vi "SendCommand_RetrieveResponse.vi"(8 "error in (no error)":errorcluster, 9 "Timeout (Seconds)":dbl=5.0 caption="Time Target (s)", 10 "Input Command":string, 11 "VISA Input":refnum<visa-resource-name>) -> (0 "error out":errorcluster, 1 "Timeout?":bool, 2 "System Response":string, 3 "VISA Output":refnum<visa-resource-name>)   [LabVIEW 2015]
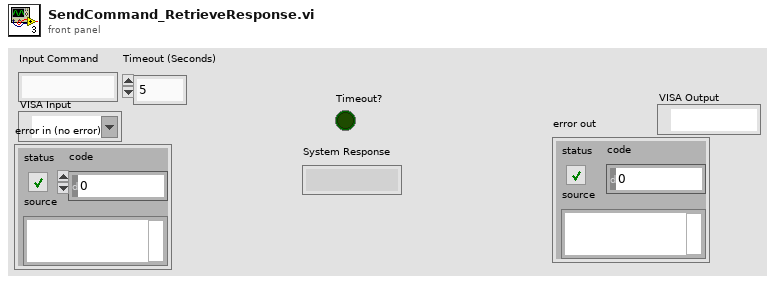
[diagram p1: front panel]
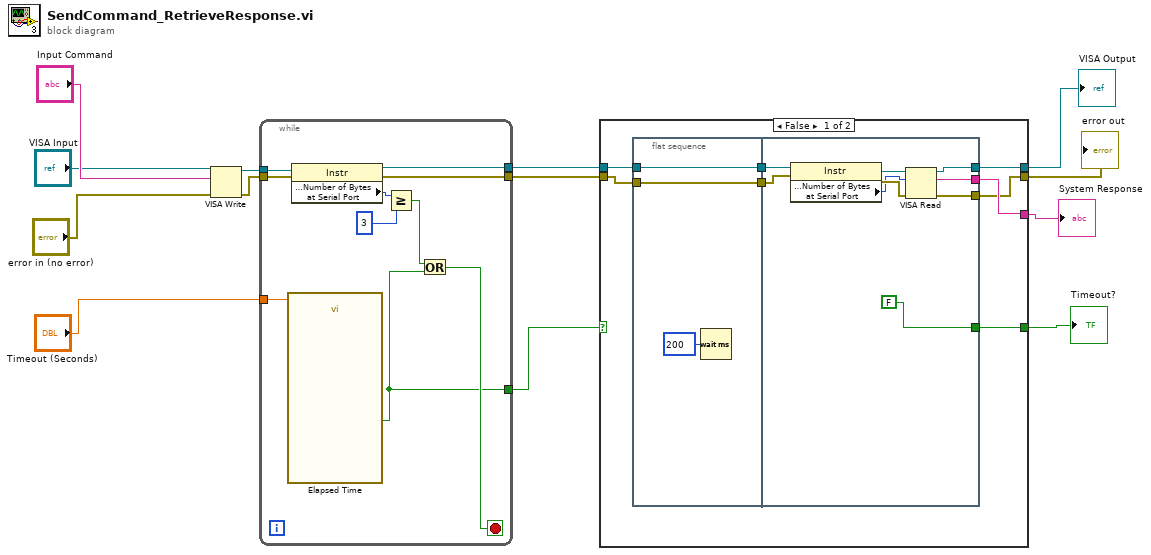
[diagram p0: block diagram]
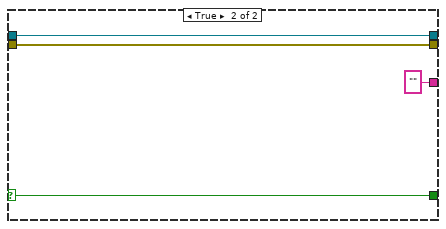
[diagram p2: hidden frame]
diagram:
  n1 = VISA Write(VISA resource name="VISA Input", write buffer="Input Command", error in (no error)="error in (no error)") -> (VISA resource name out=w13:refnum<visa-resource-name>, error out=w12:errorcluster)  [unwired: 1 out]
  n2 = while {
    tunnel: w13 -> [w23]
    tunnel: w12 -> [w22]
    tunnel: [w21] -> w6
    tunnel: [w20] -> w5
    tunnel: "Timeout (Seconds)" -> [w18]
    tunnel: [w15] -> w7
    stop <- w16 stop-if-true
    n3 = call "Elapsed Time"("Time Target (s)"=w18) -> ("Time has Elapsed"=w15:bool)  [unwired: 11 in, 7 out]
    n4 = property class="Instr"(reference=w23, error in=w22) -> (reference out=w21:refnum<visa-resource-name>, error out=w20:errorcluster, "Serial Settings:Number of Bytes at Serial Port"=w14:u32)
    n5 = Greater Or Equal?(x=w14, y=u32 3) -> (x >= y?=w17:bool)
    n6 = Or(x=w17, y=w15) -> (x .or. y?=w16:bool)
  }
  n7 = case shown="False" w7 {
    selector: w7 -> [_ w45]
    tunnel: w6 -> [w31 w47]
    tunnel: w5 -> [w30 w46]
    tunnel: [w26 w47] -> w2
    tunnel: [w25 w46] -> w1
    tunnel: [w24 w45] -> w3
    tunnel: [w27 "" ("read buffer")] -> w4
    frame False {
      n8 = flat-sequence {
        tunnel: w31 -> [w33]
        tunnel: w30 -> [w32]
        tunnel: [w33] -> w29
        tunnel: [w32] -> w28
        tunnel: w29 -> [w43]
        tunnel: w28 -> [w42]
        tunnel: [w38] -> w27
        tunnel: [w37] -> w26
        tunnel: [w36] -> w25
        tunnel: [FALSE] -> w24
        frame #0 {
          n9 = Wait (ms)(milliseconds to wait=u32 200) -> ()  [unwired: 1 out]
        }
        frame #1 {
          n10 = property class="Instr"(reference=w43, error in=w42) -> (reference out=w41:refnum<visa-resource-name>, error out=w40:errorcluster, "Serial Settings:Number of Bytes at Serial Port"=w39:u32)
          n11 = VISA Read(VISA resource name=w41, byte count=w39, error in (no error)=w40) -> (VISA resource name out=w37:refnum<visa-resource-name>, read buffer=w38:string, error out=w36:errorcluster)  [unwired: 1 out]
        }
      }
    }
    frame True {
    }
  }
  "System Response" <- w4
  "Timeout?" <- w3
  "VISA Output" <- w2
  "error out" <- w1
